vi "Get Version A.vi"() -> (3 "Version Out":string)   [LabVIEW 2018, in "labview_conan_poc_liba.lvlib"]
uses:
  labview_conan_poc_liba.lvlib
  <vilib>/Utility/LVLibp/NI_PackedLibraryUtility.lvlib
  Support/labview_conan_poc_libc.lvlibp
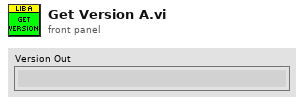
[diagram p1: front panel]
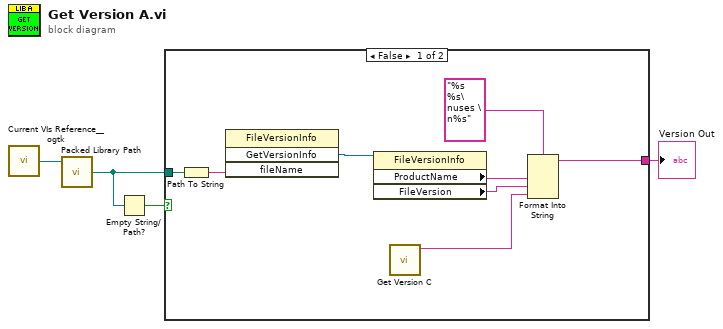
[diagram p0: block diagram]
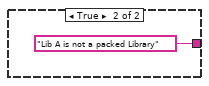
[diagram p2: hidden frame]
diagram:
  n1 = call <userlib>:"Current VIs Reference__ogtk.vi"() -> ("Current VI's reference"=w2:refnum<vi>)  [unwired: 5 in]
  n2 = call <vilib>:"Packed Library Path.vi"("vi reference"=w2) -> ("packed library path"=w4:path)  [unwired: 2 in, 2 out]
  n3 = Empty String/Path?(string/path=w4) -> (empty?=w3:bool)
  n4 = case shown="False" w3 {
    tunnel: w4 -> [w11 _]
    tunnel: [w6 "Lib A is not a packed Library"] -> w1
    frame False {
      n5 = Path To String(path=w11) -> (string=w12:string)
      n6 = invoke class="FileVersionInfo" method="GetVersionInfo"("fileName"=w12) -> ("GetVersionInfo"=w10:refnum<k24>)  [unwired: 3 in, 3 out]
      n7 = property class="FileVersionInfo"(reference=w10) -> ("ProductName"=w8:string, "FileVersion"=w7:string)  [unwired: 1 in, 2 out]
      n8 = call "Get Version C.vi"() -> ("Version Out"=w5:string)  [unwired: 11 in]
      n9 = Format Into String(format string="%s %s\nuses \n%s", w8, w7, w5) -> (resulting string=w6:string)  [unwired: 2 in, 1 out]
    }
    frame True {
    }
  }
  "Version Out" <- w1
